vi "Circular Buffer (multiple).vi"(6 "History Length [1024]":i32=1024, 7 "reset":bool, 8 "error in":errorcluster, 11 "XY-data":cluster{"X-array":dbl[], "Y-array":dbl[]}[](array[cluster]) {"Y-array" format="%.2p"; "X-array" format="%.2p"}) -> (0 "error out":errorcluster, 3 "XY-data out":cluster{"X-array":dbl[], "Y-array":dbl[]}[](array[cluster]) {"Y-array" format="%.2p"; "X-array" format="%.2p"})   [LabVIEW 2019, in "xy_utilities.lvlib"]
doc: "Circular Buffer with controllable reset and history length."
uses:
  xy_utilities.lvlib
  Typedefs/XY-Data--Cluster.ctl
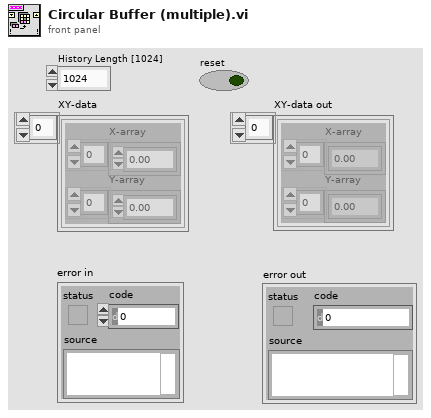
[diagram p1: front panel]
types:
  T1 = typedef "xy_utilities.lvlib/XY-Data--Cluster.ctl" = cluster{"X-array":dbl[], "Y-array":dbl[]}
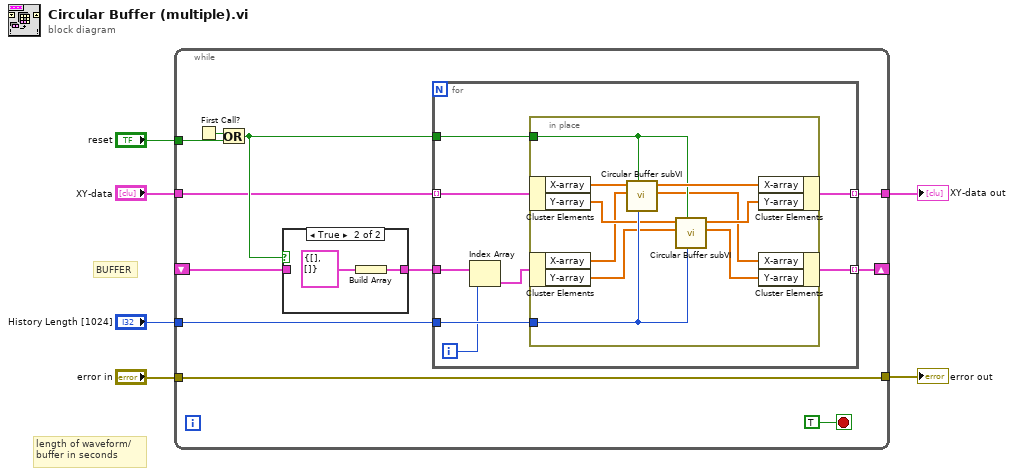
[diagram p0: block diagram]
diagram:
  # "BUFFER"
  # "length of waveform/\nbuffer in seconds"
  n1 = while {
    tunnel: "XY-data" -> [w7]
    tunnel: [w17] -> w3
    tunnel: "error in" -> [w17]
    tunnel: "reset" -> [w15]
    shift-right: [w11] -> _
    shift-left: _ -> [w9]
    tunnel: "History Length [1024]" -> [w13]
    tunnel: [w12] -> w1
    stop <- TRUE stop-if-true
    n2 = First Call?() -> (First Call?: T/F=w16:bool)
    n3 = Or(x=w16, y=w15) -> (x .or. y?=w8:bool)
    n4 = case shown="True" w8 {
      tunnel: w9 -> [w36 _]
      tunnel: [w36 w37] -> w10
      frame False {
      }
      frame True {
        n5 = Build Array(T1 {"X-array"=[], "Y-array"=[]} ("XY-data")) -> (w37:T1[])
      }
    }
    n6 = for {
      tunnel: w13 -> [w25]
      tunnel: [w24] -> w12 mode=indexing
      tunnel: [w23] -> w11 mode=indexing
      tunnel: w10 -> [w18]
      tunnel: w7 -> [w22] mode=indexing
      tunnel: w8 -> [w21]
      i -> [w20]
      n7 = Index Array(array=w18, index=w20) -> (element=w19:T1)
      n8 = in-place {
        in-place-border: w25 -> [w32]
        in-place-border: w21 -> [w33]
        n9 = in-place-cluster #1(w22) -> ("X-array"=w35:dbl[], "Y-array"=w30:dbl[])
        n10 = in-place-cluster #2(w19) -> ("X-array"=w29:dbl[], "Y-array"=w26:dbl[])
        n11 = call "Circular Buffer subVI.vi"("History Length [1024]"=w32, "Reset"=w33, "Buffer in"=w29, "Array in"=w35) -> ("Buffer out"=w27:dbl[], "Array out"=w34:dbl[])  [unwired: 6 in]
        n12 = call "Circular Buffer subVI.vi"("History Length [1024]"=w32, "Reset"=w33, "Buffer in"=w26, "Array in"=w30) -> ("Buffer out"=w28:dbl[], "Array out"=w31:dbl[])  [unwired: 6 in]
        n13 = in-place-cluster #1("X-array"=w34, "Y-array"=w31) -> (w24:cluster{"X-array":dbl[], "Y-array":dbl[]})
        n14 = in-place-cluster #2("X-array"=w27, "Y-array"=w28) -> (w23:T1)
      }
    }
  }
  "XY-data out" <- w1
  "error out" <- w3
